vi "Flush Data to Offsite Log Bin File.vi"(0 "Logging Configuration":T1, 1 "Data Queue":refnum<queue>, 3 "error in (no error)":errorcluster) -> (10 "error out":errorcluster)   [LabVIEW 2017, in "Logging.lvlib"]
uses:
  Logging.lvlib
  Logging Configuration.ctl
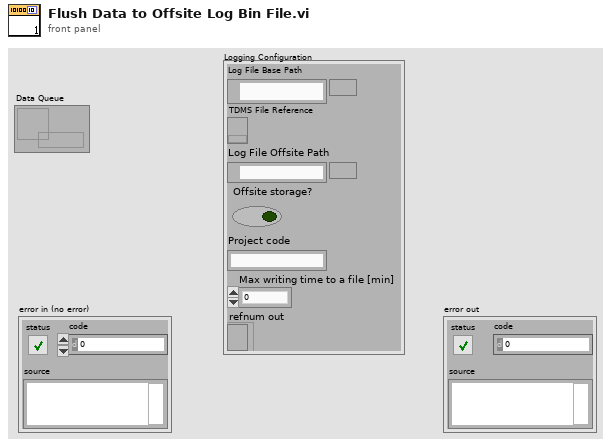
[diagram p1: front panel]
types:
  T1 = typedef "Logging.lvlib/Logging Configuration.ctl" = cluster{"Log File Base Path":path, "TDMS File Reference":refnum<k34>, "Log File Offsite Path":path, "Offsite storage?":bool, "Project code":string, "Max writing time to a file [min]":dbl, "refnum out":refnum<file>}
  T2 = enum16{"big-endian, network order", "native, host order", "little-endian"}
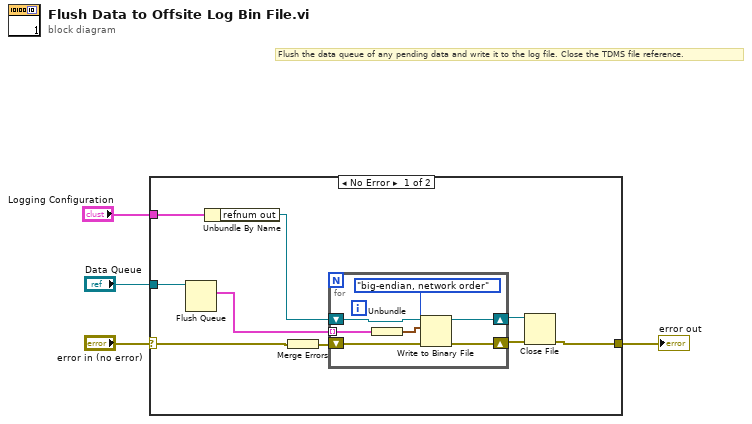
[diagram p0: block diagram]
diagram:
  # "Flush the data queue of any pending data and write it to the log file. Close the TDMS file reference."
  n1 = case shown="No Error" "error in (no error)" {
    selector: "error in (no error)" -> [w9 w21]
    tunnel: "Data Queue" -> [w11 _]
    tunnel: [w10 w21] -> w3
    tunnel: "Logging Configuration" -> [w6 _]
    frame No Error {
      n2 = Flush Queue(queue=w11) -> (remaining elements=w13:cluster{"Array":waveform(dbl)[]}[])  [unwired: 1 in, 2 out]
      n3 = Unbundle By Name(w6) -> ("refnum out"=w5:refnum<file>)
      n4 = Merge Errors(w9) -> (w8:errorcluster)
      n5 = for {
        shift-right: [w15] -> w7
        shift-left: w5 -> [w16]
        shift-right: [w19] -> w12
        shift-left: w8 -> [w20]
        tunnel: w13 -> [w18] mode=indexing
        n6 = Unbundle(w18) -> ("Array"=w17:waveform(dbl)[])
        n7 = Write to Binary File(file (use dialog)=w16, data=w17, error in=w20, 9:T2."big-endian, network order" ("byte order (0:big-endian, network order)")) -> (refnum out=w15:refnum<file>, error out=w19:errorcluster)  [unwired: 2 in, 1 out]
      }
      n8 = Close File(refnum=w7, error in=w12) -> (error out=w10:errorcluster)  [unwired: 1 out]
    }
    frame Error {
    }
  }
  "error out" <- w3
